vi "initialize digestsign.vi"(8 "error in":errorcluster, 10 "pkey":u64, 11 "digest name":string) -> (0 "error out":errorcluster, 3 "lvlibcrypto digest out":refnum<class "lvlibcrypto digestsign.lvclass">)   [LabVIEW 2016, in "lvlibcrypto digestsign.lvclass"]
uses:
  lvlibcrypto digestsign.lvclass
  lvlibcrypto digestsign.lvclass/lvlibcrypto digestsign.ctl
  lv tls dll.lvlib
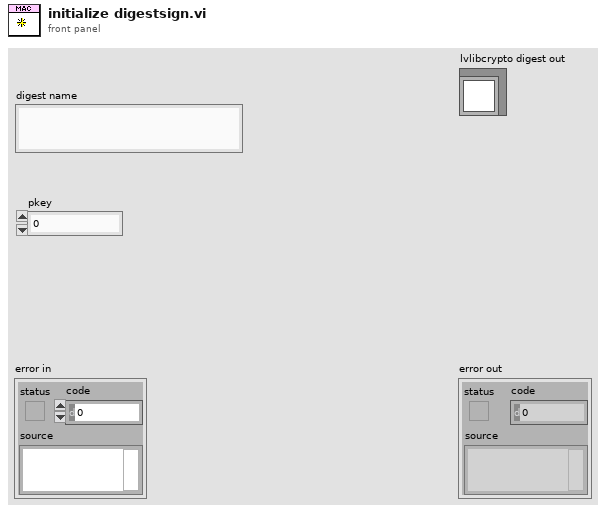
[diagram p1: front panel]
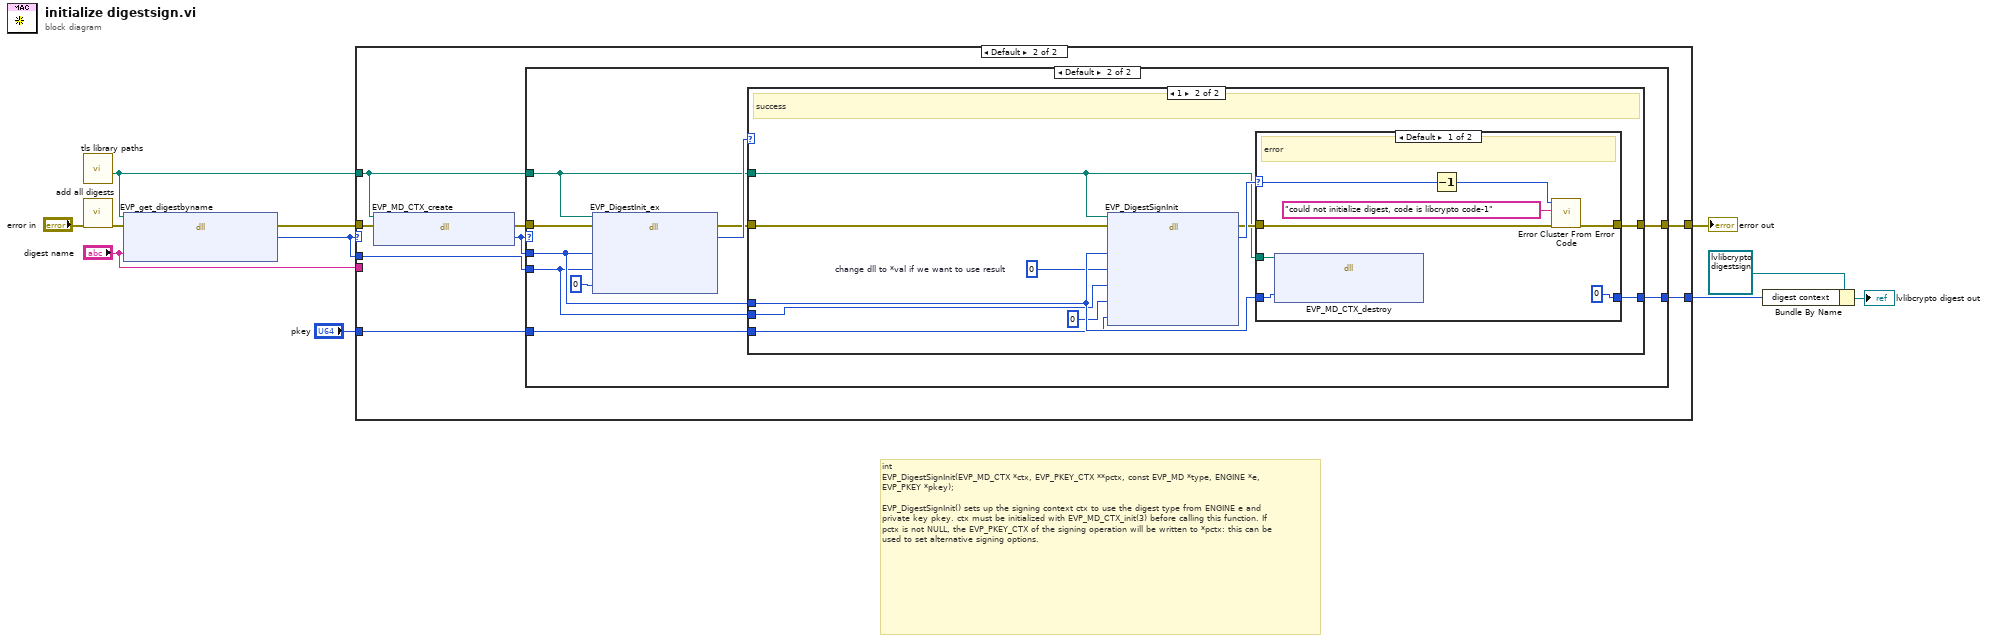
[diagram p0: block diagram]
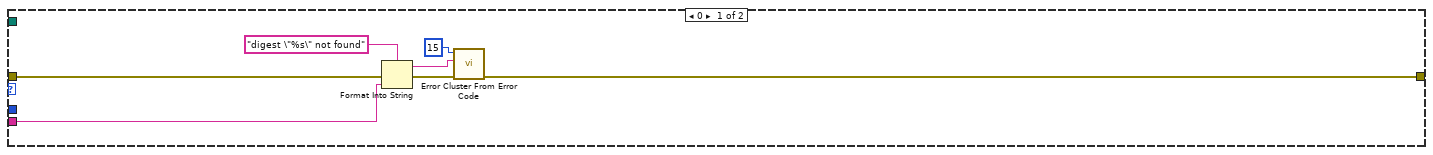
[diagram p2: hidden frame]
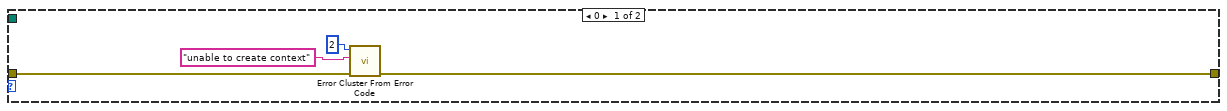
[diagram p3: hidden frame]
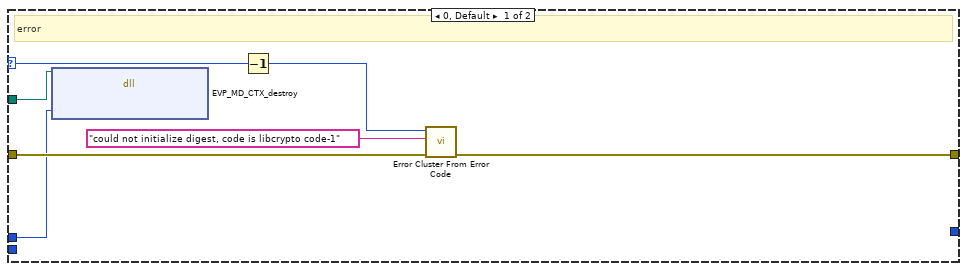
[diagram p4: hidden frame]
diagram:
  # "int \nEVP_DigestSignInit(EVP_MD_CTX *ctx, EVP_PKEY_CTX **pctx, const EVP_MD *type, ENGINE *e, EVP_PKEY *pkey);\n\nEVP_DigestSignInit() sets up the signing context ctx to use the digest type from ENGINE e and private key pkey. ctx must be initialized with EVP_MD_CTX_init(3) before calling this function. If pctx is not NULL, the EVP_PKEY_CTX of the signing operation will be written to *pctx: this can be used to set alternative signing options."
  n1 = call "tls library paths.vi"() -> ("libcrypto"=w4:path)  [unwired: 8 in, 3 out]
  n2 = call "add all digests.vi"("error in"="error in") -> ("error out"=w2:errorcluster)  [unwired: 10 in]
  n3 = dll-call lib="C:/Users/IEUser/Desktop/tlssimple/libcrypto-41.dll" fn="EVP_get_digestbyname"(path in=w4, error in=w2, "digestname"="digest name") -> (error out=w10:errorcluster, "md"=w7:u64)  [unwired: 2 in, 1 out]
  n4 = case shown="Default" w7 {
    tunnel: w10 -> [w18 w19]
    tunnel: w4 -> [_ w22]
    tunnel: [w17 w25] -> w9
    tunnel: "digest name" -> [w13 _]
    tunnel: w7 -> [_ w21]
    tunnel: [_ w23] -> w5
    tunnel: "pkey" -> [_ w20]
    frame 0 {
      n5 = Format Into String(format string="digest \"%s\" not found", error in=w18, w13) -> (resulting string=w14:string, error out=w15:errorcluster)  [unwired: 1 in]
      n6 = call <vilib>:"Error Cluster From Error Code.vi"("error in (no error)"=w15, "error message (\"\")"=w14, "error code (0)"=15) -> ("error out"=w17:errorcluster)  [unwired: 6 in]
    }
    frame Default {
      n7 = dll-call lib="C:/Users/IEUser/Desktop/tlssimple/libcrypto-41.dll" fn="EVP_MD_CTX_create"(path in=w22, error in=w19) -> (error out=w26:errorcluster, "context"=w24:u64)  [unwired: 1 in, 1 out]
      n8 = case shown="Default" w24 {
        tunnel: w26 -> [w30 w40]
        tunnel: [w29 w37] -> w25
        tunnel: w24 -> [_ w34]
        tunnel: w21 -> [_ w31]
        tunnel: w22 -> [_ w35]
        tunnel: [_ w33] -> w23
        tunnel: w20 -> [_ w32]
        frame 0 {
          n9 = call <vilib>:"Error Cluster From Error Code.vi"("error in (no error)"=w30, "error message (\"\")"="unable to create context" ("error message (\"\")"), "error code (0)"=2) -> ("error out"=w29:errorcluster)  [unwired: 6 in]
        }
        frame Default {
          n10 = dll-call lib="C:/Users/IEUser/Desktop/tlssimple/libcrypto-41.dll" fn="EVP_DigestInit_ex"(path in=w35, error in=w40, "context"=w34, "digesttype"=w31, "engine null"=u64 0) -> (error out=w36:errorcluster, "ret"=w38:i32)  [unwired: 4 in, 1 out]
          n11 = case shown="1" w38 {
            selector: w38 -> [w45 _]
            tunnel: [w46 w56] -> w37
            tunnel: w36 -> [w47 w58]
            tunnel: w35 -> [w42 w52]
            tunnel: w34 -> [w41 w53]
            tunnel: [_ w54] -> w33
            tunnel: w32 -> [_ w49]
            tunnel: w31 -> [_ w48]
            frame 0, Default {
              # "error"
              n12 = dll-call lib="C:/Users/IEUser/Desktop/tlssimple/libcrypto-41.dll" fn="EVP_MD_CTX_destroy"(path in=w42, "context"=w41) -> ()  [unwired: 4 in, 2 out]
              n13 = Decrement(x=w45) -> (x-1=w44:i32)
              n14 = call <vilib>:"Error Cluster From Error Code.vi"("error in (no error)"=w47, "error message (\"\")"="could not initialize digest, code is libcrypto code-1" ("error message (\"\")"), "error code (0)"=w44) -> ("error out"=w46:errorcluster)  [unwired: 6 in]
            }
            frame 1 {
              w51 = 0  # change dll to *val if we want to use result
              # "success"
              n15 = dll-call lib="C:/Users/IEUser/Desktop/tlssimple/libcrypto-41.dll" fn="EVP_DigestSignInit"(path in=w52, error in=w58, "context"=w53, "pkcontext"=w51, "digesttype"=w48, "engine null"=u64 0, "pkey"=w49) -> (error out=w55:errorcluster, "ret"=w57:i32)  [unwired: 6 in, 1 out]
              n16 = case shown="Default" w57 {
                selector: w57 -> [w61 _]
                tunnel: [w62 w68] -> w56
                tunnel: w55 -> [w63 w68]
                tunnel: [u64 0 ("context") w67] -> w54
                tunnel: w53 -> [w66 w67]
                tunnel: w52 -> [w59 _]
                frame Default {
                  # "error"
                  n17 = dll-call lib="C:/Users/IEUser/Desktop/tlssimple/libcrypto-41.dll" fn="EVP_MD_CTX_destroy"(path in=w59, "context"=w66) -> ()  [unwired: 4 in, 2 out]
                  n18 = Decrement(x=w61) -> (x-1=w65:i32)
                  n19 = call <vilib>:"Error Cluster From Error Code.vi"("error in (no error)"=w63, "error message (\"\")"="could not initialize digest, code is libcrypto code-1" ("error message (\"\")"), "error code (0)"=w65) -> ("error out"=w62:errorcluster)  [unwired: 6 in]
                }
                frame 1 {
                  # "success"
                }
              }
            }
          }
        }
      }
    }
  }
  "error out" <- w9
  n20 = Bundle By Name(cluster=refnum<class "lvlibcrypto digestsign.lvclass"> refnum ("lvlibcrypto digest in"), "digest context"=w5) -> (→"lvlibcrypto digest out":refnum<class "lvlibcrypto digestsign.lvclass">)
